vi "Dashboard Main.vi"() -> ()   [LabVIEW 2025]
uses:
  builds/FRC_Dashboard/data/Bordeaux/Types/Single Cmd Info.ctl
  <vilib>/picture/picture.llb/imagedata.ctl
  <vilib>/Rock Robotics/WPI/DriverStation/WPI_DriverStationAllianceInfo.ctl
  <vilib>/Utility/miscctls.llb/LVPoint32TypeDef.ctl
  builds/FRC_Dashboard/data/Bordeaux/Types/Drive Type.ctl
  52f2dcef-b32f-41dc-9262-467f65fbdc6c.vi
  builds/FRC_Dashboard/data/Bordeaux/Global Settings.vi
  <vilib>/Rock Robotics/Network Tables/NT Write String Array.vi
  <vilib>/Rock Robotics/WPI/Dashboard/WPI_DashboardLogging Global.vi
  <vilib>/Rock Robotics/Network Tables/NT Write Number.vi
  <vilib>/Rock Robotics/Network Tables/NT Write Boolean.vi
  <vilib>/Rock Robotics/Network Tables/NT Read Integer.vi
  <vilib>/Rock Robotics/Network Tables/NT Read Number.vi
  <vilib>/Rock Robotics/Network Tables/NT Read Numeric Array.vi
  <vilib>/ErrorRing/Error Ring.xnode
  <vilib>/MakerHub/Toolbox/LMH-Toolbox.lvlib
panel:
  out "path":string[](array[string])
  out "ACTIVITY STATUS":dbl[][](graph)
  in  "Camera Settings Right":T1={"Frame Rate"=30, "Compression"=30, "Size"=1, "DB Camera Config"=FALSE} {"Frame Rate" scale=1.0..30.0; "Compression" scale=100.0..-1.0; "Size" items=["640x480", "320x240", "160x120"]}
  in  "Camera Name Right":string(combo)="No Camera Selection"
  out "NT Connection":bool
  in  "Camera Settings":T1={"Frame Rate"=30, "Compression"=30, "Size"=1, "DB Camera Config"=FALSE} {"Frame Rate" scale=1.0..30.0; "Compression" scale=100.0..-1.0; "Size" items=["640x480", "320x240", "160x120"]}
  in  "Camera Name":string(combo)="No Camera Selection"
  in  "TCP":refnum<k5>
  in  "Rec Mode":enum32{"Stop", "Record", "Playback"}(radio)
  out "Robot IP":string
  out "Image Message":string="Timeout in Camera Communications"
  in  "Dashboard Tab":T2(tab)
  in  "Offset":dbl=270.0
  out "Boolean 2":bool
  in  "Active Status":bool
  out "Boolean":bool
  out "Picture":picture
  in  "Auto Delay?":bool
  in  "Delay Time (s)":dbl
  in  "Aquitaine File":string
  in  "Auto Calibrate":bool=TRUE
  in  "Manual Paths":string[](array[string])
  in  "Max Rotation":dbl=270.0
  in  "Max Translation":dbl=19.0
  in  "Deadband":dbl=0.05
  in  "Auto Selector":T3(ring)
  out "IMU":dbl(knob) scale=-180.0..180.0
  in  "Select Auto":string(combo)="Select Autonomous ..."
  out "Mode":T4(ring)=enum."Auto Disabled"
  out "Camera Perf":cluster{"Bandwidth (Mbps)":dbl, "FPS":dbl}
  out "Camera Perf 2":string
  out "Auto Picture":picture
  out "path info":string
  in  "restart":bool
  out "Picture 2":picture
  out "Camera Perf 3":string
  out "DISTANCE":dbl
  out "PTH":dbl(knob) scale=-180.0..180.0
  out "Tree":string(tree)
  # "HW"
  # "HW"
  # "IMU"
  # "SWERVE"
  # "AUTONOMOUS"
  # "CONFIGS"
  # "TAG VISIBILITY"
  # "STATUS"
  # "PLACEHOLDER"
  # "PLACEHOLDER"
  # "CAN ERROR"
  # "SENSOR FAULT"
  # "GATE DRIVER"
  # "No POWER"
  # "Full FORWARD"
  # "Full REVERSE"
  # "BRUSHED BRAKE"
  # "BRUSHED COAST"
  # "BRUSHLESS BRAKE"
  # "BRUSHLESS COAST"
  # "RECOVERY MODE/OFF"
  # "https://cdn8.bigcommerce.com/s-t3eo8vwp22/product_images/uploaded_images/fault-no-12v.gif"
  # "PIGEON 2"
  # "DAMAGED HARDWARE"
  # "BOOTLOADER"
  # "CAN FAULT"
  # "ROBOT DISABLED"
  # "ROBOT ENABLED"
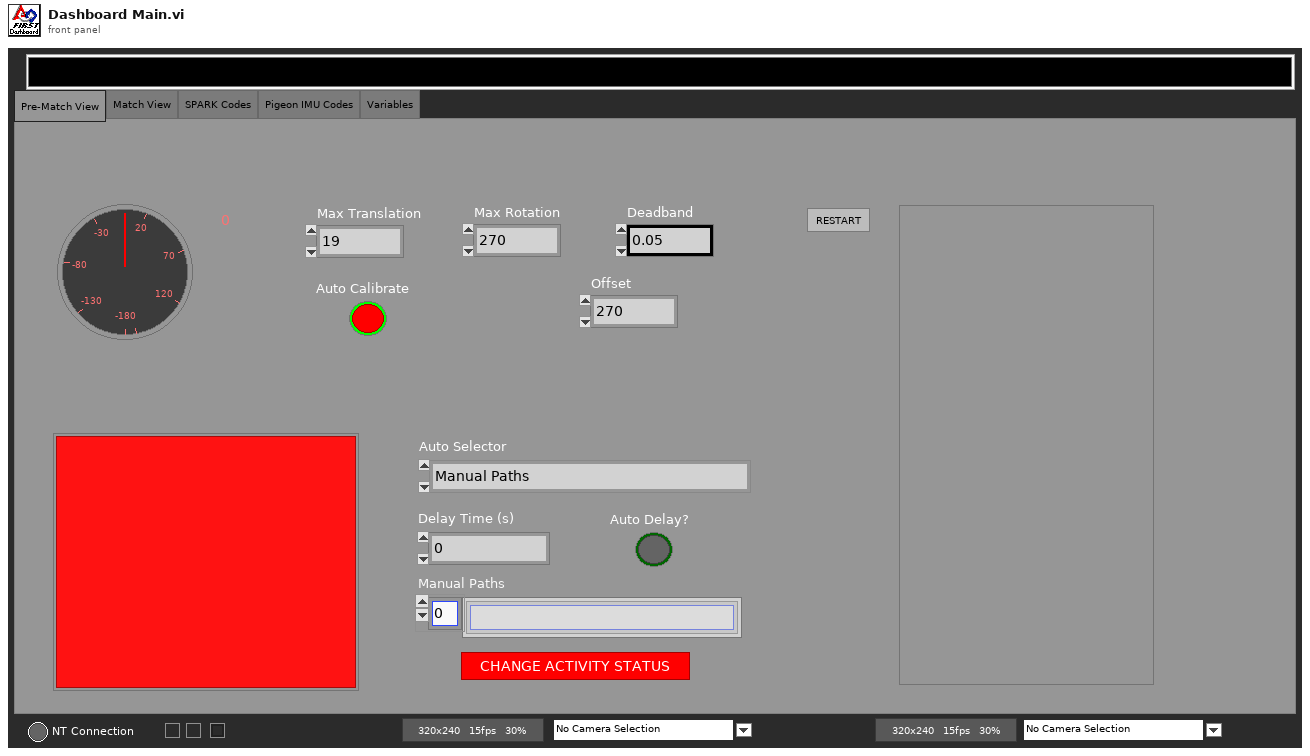
[diagram p1: front panel]
types:
  T1 = cluster{"Frame Rate":i32, "Compression":i32, "Size":u16, "DB Camera Config":bool}
  T2 = enum32{"Pre-Match View", "Match View", "SPARK Codes", "Pigeon IMU Codes", "Variables"}
  T3 = enum16{"Manual Paths", "Custom Paths", "Red Right Neutral", "Blue Right Neutral", "Red Left Neutral", "Blue Left Neutral", "Red Right 86 ", "Blue Right 86", "Red Left 86", "Blue Left 86"}
  T4 = enum8{"Tele-Op Disabled", "Tele-Op Enabled", "Auto Disabled", "Auto Enabled", "Test Disabled", "Test Enabled", "Disconnected", "No Code", "E-Stop"}
  T5 = cluster{"Save Path":path, "Interval (s)":dbl, "Keep":i32}
  T6 = typedef "Image Type" = u32
  T7 = enum32{"Pre-Match View", "Match View", "SparkMax Codes", "Pigeon IMU Codes", "Variables"}
  T8 = cluster{"IDs":cluster{"RPC field ID":u16, "Unique ID":u16}, "String":string}
  T9 = typedef "IMAQ Image.ctl" = refnum<image>
  T10 = cluster{"Dashboard Tab":refnum<vi>, "Rec Mode":refnum<vi>, "Tree":refnum<vi>, "Camera Perf 2":refnum<vi>, "Camera Settings":refnum<vi>, "Camera Name":refnum<vi>, "Camera Name":refnum<vi>}
  T11 = cluster{"Camera Name Right":string, string, "Saved DB Images Info":cluster{"Save Path":path, "Interval (s)":dbl, "Keep":i32}}
  T12 = cluster{"Global Rectangle":i32[], "Contours":cluster{"Contour Type":u32, "ROI Type":u32, "Points":i32[]}[]}
  T13 = cluster{"Camera Name":string, string, "Saved DB Images Info":cluster{"Save Path":path, "Interval (s)":dbl, "Keep":i32}}
  T14 = typedef "Single Cmd Info.ctl" = cluster{"Name":string, "CPTM.DataType":variant, "All Control Values Variant":cluster{"Name":string, "Variant Data":variant}[], "icon full":T15, "icon scaled":T15, "Path":path, "Subsystem Color":u32}
  T15 = typedef "imagedata.ctl" = cluster{"image type":i32, "image depth":i32, "image":u8[], "mask":u8[], "colors":u32[], "Rectangle":cluster{"left":i16, "top":i16, "right":i16, "bottom":i16}}
  T16 = typedef "Drive Type.ctl" = enum16{"Nonholonomic", "Holonomic"}
  T17 = typedef "LVPoint32TypeDef.ctl" = cluster{"Horizontal":i32, "Vertical":i32}
  T18 = cluster{"Index":i32, "Pt Test Results":enum16{"Miss", "Rect Hit", "Arrow Hit"}}
  T19 = cluster{"Error Strings":string, "Disable Counts":cluster{u16, u16}, "Rail Faults":cluster{u16, u16, u16}, "Robot IP":string, "DB Mode":u8, "Event Info":cluster{"Name":string, "Type":u8, "Number":u16, "Replay":u8}}
  T20 = cluster{"Storage":cluster{"Disk Free":u64, "RAM Block":u32, "RAM free":u32}, "CPU Utilization":cluster{"CPU % ISR":sgl, "CPU % Time Crit":sgl, "CPU % Timed Str":sgl, "CPU % High":sgl, "CPU % Above":sgl, "CPU % Normal":sgl, "CPU % Low":sgl}, "CAN":cluster{"% Bus Utilization":sgl, "Bus Off Cnt":u32, "TX_FIFO Full Cnt":u32, "Receive Error Cnt":u8, "Transmit Error Cnt":u8}, "HID":cluster{"HID Outputs":u32, "Rumble Low":u16, "Rumble High":u16}[]}
  T21 = cluster{"Status bits":cluster{"Test Mode":bool, "Autonomous":bool, "Enabled":bool, "Code Start":bool, "Brownout":bool, "Reserved 2":bool, "Reserved 3":bool, "E-Stop":bool}, "Code Trace":cluster{"Disabled":bool, "TeleOp":bool, "Auto":bool, "Test":bool}, "Controller Type":enum16{"unknown", "cRIO", "roboRio"}, "Code?":enum16{"unknown", "noCode", "code"}, "Battery V":dbl}
  T22 = cluster{"Control Bits":cluster{"TestMode":bool, "Autonomous":bool, "Enabled":bool, "FMS Present":bool, bool, bool, bool, "E-Stop":bool}, "Team Station ":u8, "Countdown":sgl, "Joystick Values":cluster{"Axes":dbl[], "Buttons":bool[], "POVs":i16[]}[]}
  T23 = cluster{"Robot Backwards":bool, "Reverse Path":bool}
  T24 = typedef "Trajectory Data.ctl" = cluster{"Segment Name":string, "Type":T25, "Traj Pos Points":cluster{"x":dbl, "y":dbl, "th":dbl}[], "Traj Vel Points":cluster{"V":dbl, "Omega":dbl, "V vector":cluster{"y":dbl, "x":dbl}}[], "Accel Index":i32, "Decel Index":i32}[]
  T25 = typedef "Segment Type.ctl" = enum16{"Accel Straight", "Const Straight", "Blend", "Circle", "Bezier"}
  T26 = typedef "Overrides.ctl" = cluster{"Count":string, "Angular Override":dbl, "Enabled?":bool, "Velocity Override":dbl, "Angle Override":dbl}[]
  T27 = typedef "Angluar Limits.ctl" = cluster{"Velocity (deg/s)":dbl, "Accel (deg/s^2)":dbl, "Jerk (deg/s^3)":dbl}
  T28 = cluster{"Sample Period (s)":dbl, cluster{"Velocity (fps)":dbl, "Accel (fps^2)":dbl, "Jerk (fps^3)":dbl, "StoopidFast (fps)":dbl}, "Conditions":cluster{"vInitial (fps)":dbl, "vFinal (fps)":dbl}, "Overrides":T26, "Angular Limits":T27}
  T29 = typedef "Path Type.ctl" = enum16{"Clothoid", "Bezier"}
  T30 = cluster{"status":bool, "code":bool, "source":bool}
  T31 = cluster{"Reversals":cluster{"Robot Backwards":bool, "Reverse Path":bool}, "Trajectory Data":T24, "Commands out":cluster{"Time (s)":dbl, T14, bool}[], "Fields":cluster{"Sample Period (s)":dbl, cluster{"Velocity (fps)":dbl, "Accel (fps^2)":dbl, "Jerk (fps^3)":dbl, "StoopidFast (fps)":dbl}, "Conditions":cluster{"vInitial (fps)":dbl, "vFinal (fps)":dbl}, "Overrides":T26, "Angular Limits":T27}, "Points out":cluster{"x":dbl, "y":dbl, "th":dbl}[], "Overall":cluster{"Time (s)":dbl, "Distance (ft)":dbl}, "Zero V":bool, "Trajectory Meta":cluster{"Drive Type":T16, "Path Type":T29}}
  T32 = typedef "MEGA traj.ctl" = cluster{cluster{"Robot Backwards":bool, "Reverse Path":bool}, "Trajectory Data":T24, "sorted array out":cluster{"Time (s)":dbl, T14, bool}[], cluster{"Sample Period (s)":dbl, "Limits":T33, "Conditions":cluster{"vInitial (fps)":dbl, "vFinal (fps)":dbl}, "Overrides":T26, "Angular Limits":T27}, "Updated Waypoints":cluster{"x":dbl, "y":dbl, "th":dbl}[], cluster{"Time (s)":dbl, "Distance (ft)":dbl}, "Zero Velocity":bool, cluster{"Drive Type":T16, "Path Type":T29}}[]
  T33 = typedef "Limits.ctl" = cluster{"Velocity (fps)":dbl, "Accel (fps^2)":dbl, "Jerk (fps^3)":dbl, "StoopidFast (fps)":dbl}
  T34 = cluster{"Horizontal":dbl, "Vertical":dbl, "th":dbl}
  T35 = cluster{"Horizontal":dbl, "Vertical":dbl, "th":dbl}[]
  T36 = cluster{"Operation":enum16{"Update", "Clear"}, "Color Box":u32}[]
  T37 = cluster{"Image Size":bool, "Image Type":bool, "Pixel Value":bool, "ROI Information":bool, "Zoom Factor":bool}
  T38 = cluster{"Shift":bool, "Ctrl":bool, "Alt":bool, "Cmd":bool, "Opt":bool}
  T39 = typedef "WPI_DriverStationAllianceInfo.ctl" = enum16{"Red", "Blue", "Invalid"}
  T40 = cluster{"Numeric":dbl, "Numeric":dbl, "Numeric":dbl}
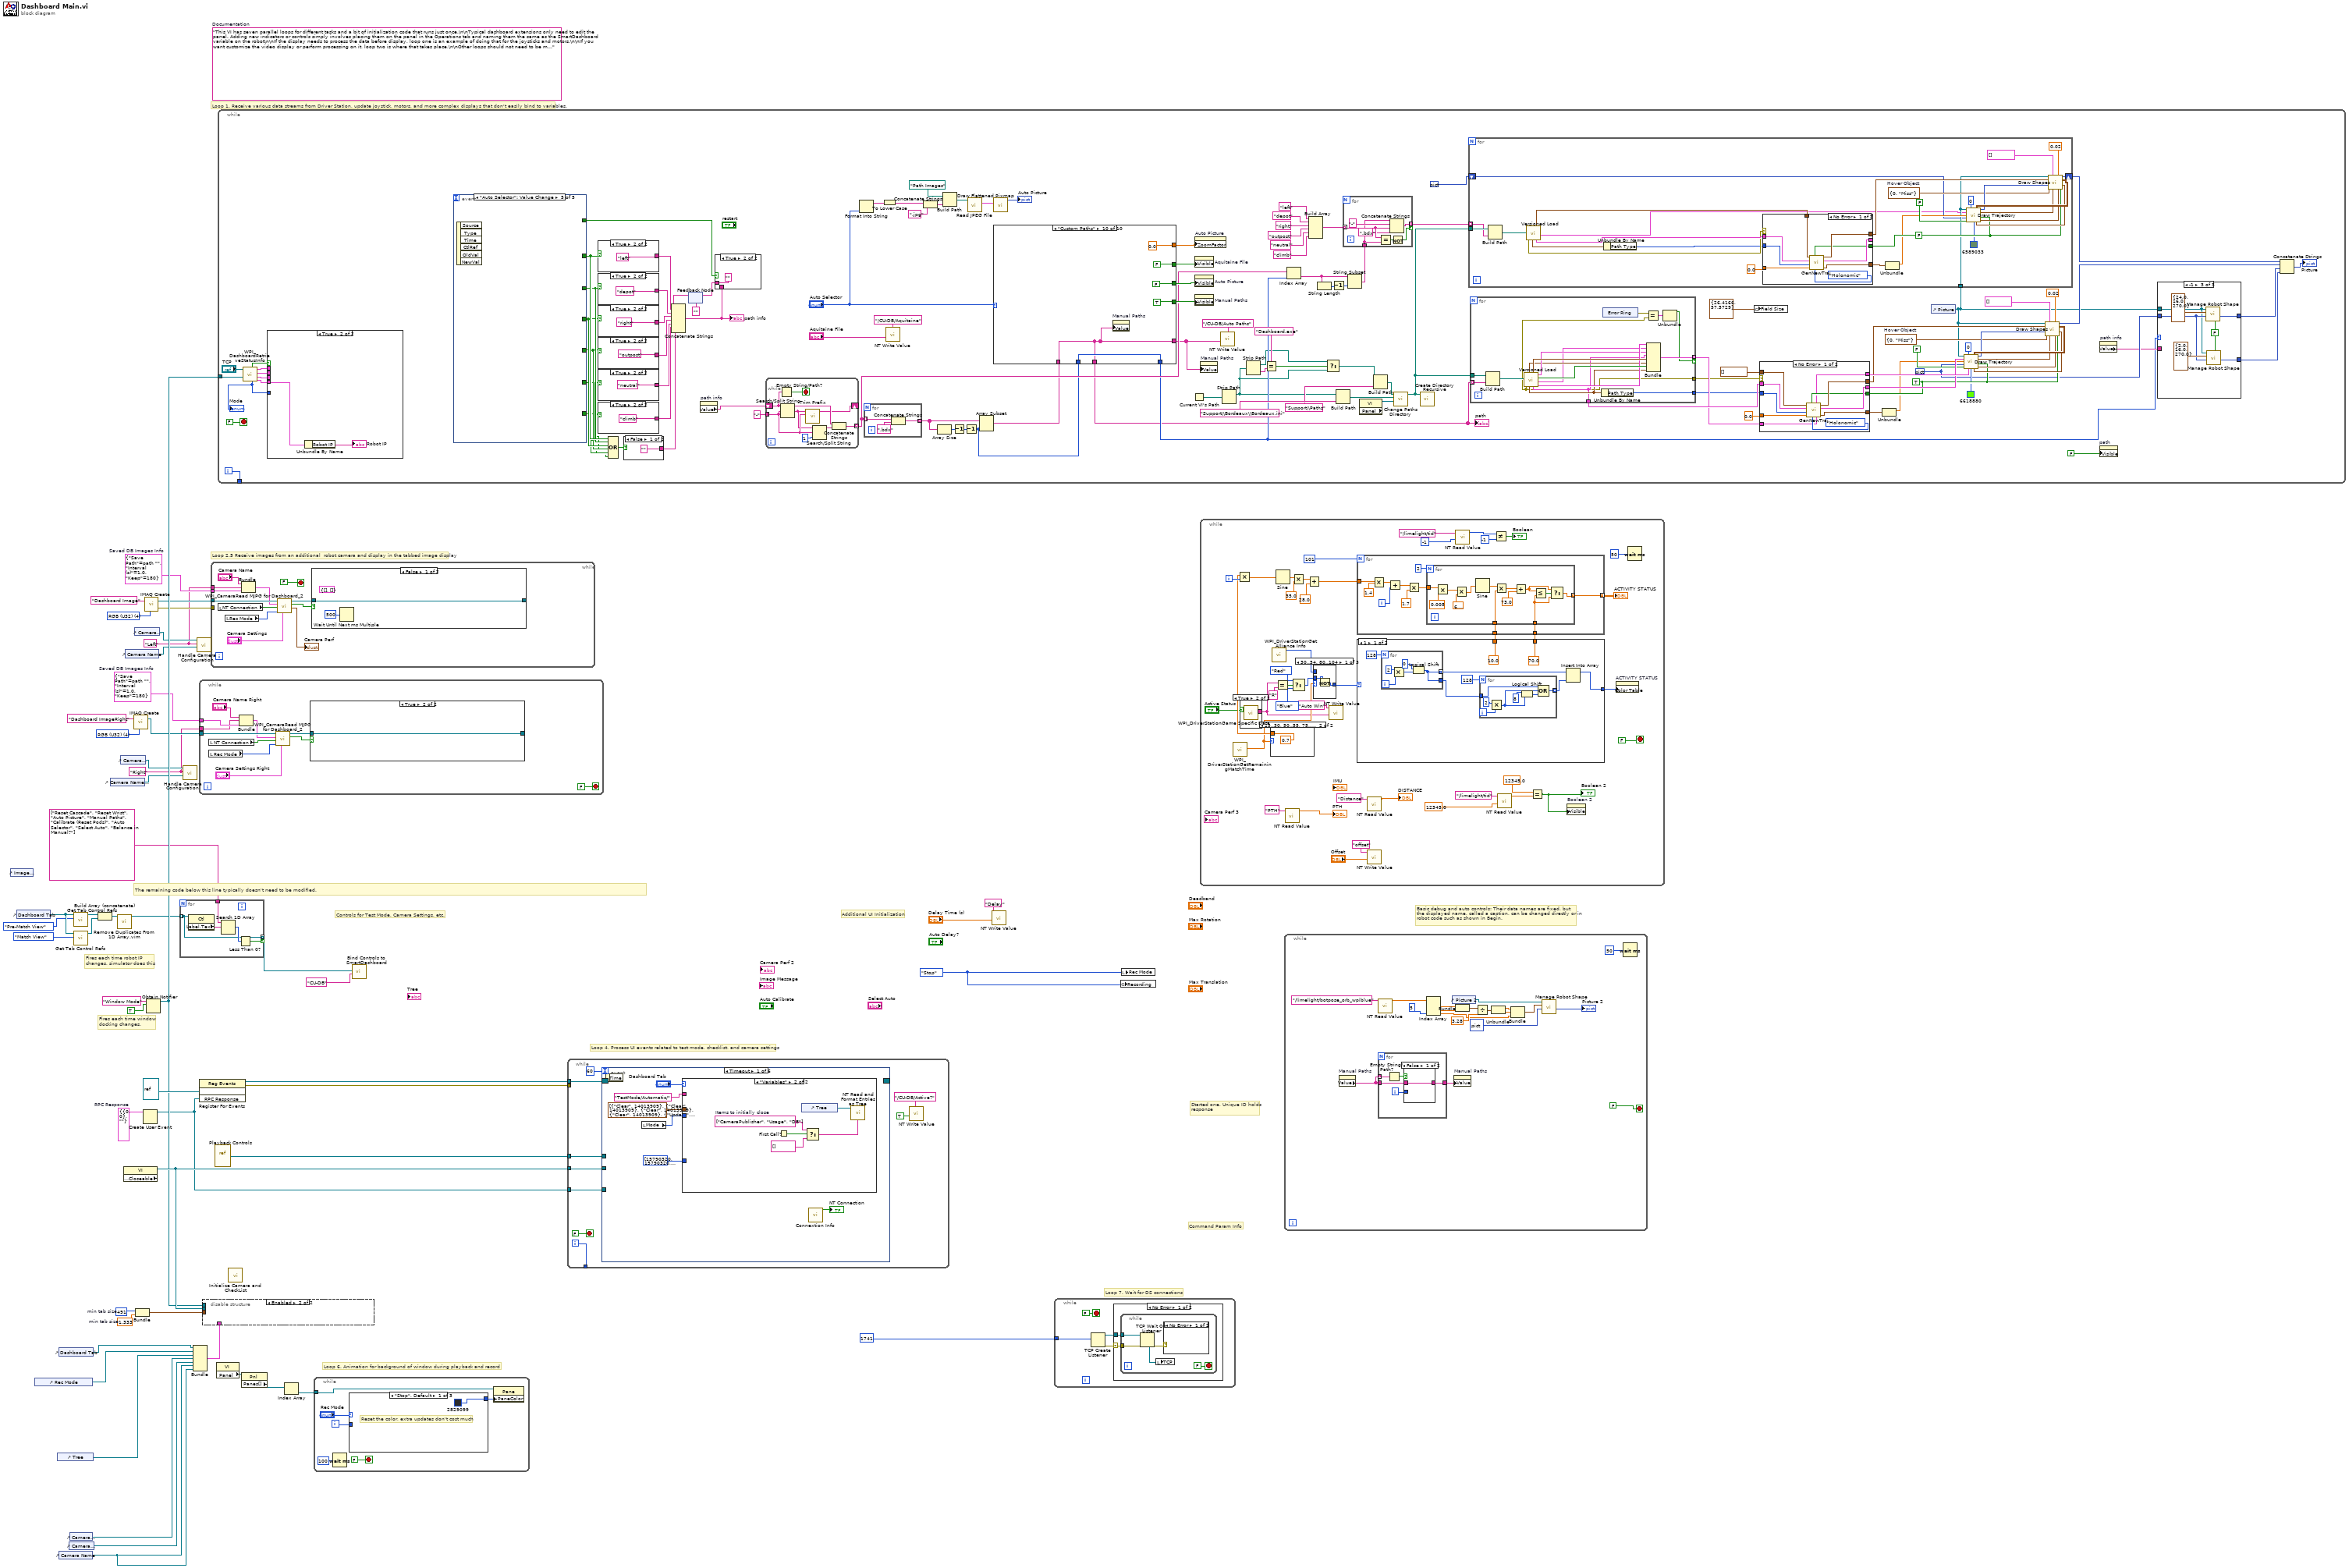
[diagram p0: block diagram]
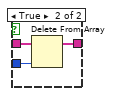
[diagram p2: hidden frame]
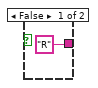
[diagram p3: hidden frame]
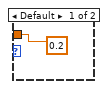
[diagram p6: hidden frame]
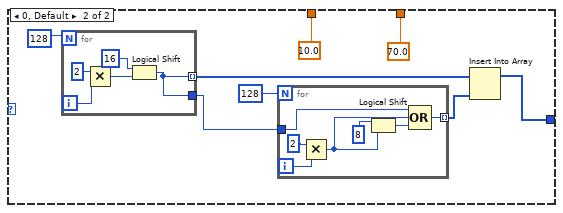
[diagram p7: hidden frame]
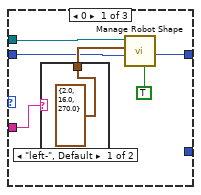
[diagram p8: hidden frame]
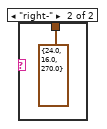
[diagram p9: hidden frame]
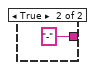
[diagram p13: hidden frame]
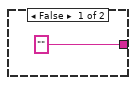
[diagram p14: hidden frame]
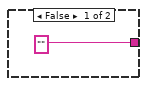
[diagram p15: hidden frame]
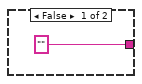
[diagram p16: hidden frame]
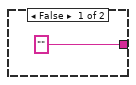
[diagram p17: hidden frame]
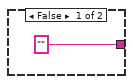
[diagram p18: hidden frame]
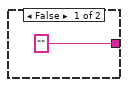
[diagram p19: hidden frame]
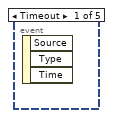
[diagram p20: hidden frame]
diagram:
  w4 = "Right"
  w9 = T5 {"Save Path"=path "", "Interval (s)"=1.0, "Keep"=180}  # Saved DB Images Info
  w11 = T6 4 items=["Grayscale (U8)", "Grayscale (I16)", "Grayscale (SGL)", "Complex (CSG)", "RGB (U32)", "HSL (U32)", "RGB (U64)"] ("Image Type")
  w27 = T5 {"Save Path"=path "", "Interval (s)"=1.0, "Keep"=180}  # Saved DB Images Info
  w8 = "Left"
  w30 = T6 4 items=["Grayscale (U8)", "Grayscale (I16)", "Grayscale (SGL)", "Complex (CSG)", "RGB (U32)", "HSL (U32)", "RGB (U64)"] ("Image Type")
  w34 = T8 {"IDs"={"RPC field ID"=0, "Unique ID"=0}, "String"=""}  # RPC Response
  w41 = 491  # min tab size
  w40 = 1.333  # min tab size
  w43 = enum32{"Stop", "Record", "Playback"}."Stop" ("Rec Mode")
  (unwired) "This VI has seven parallel loops for different tasks and a bit of initialization code that runs just once.\n\nTypical dashboard extensions only need to edit the panel. Adding new indicators or controls simply involves placing them on the panel in the Operations tab and naming them the same as the SmartDashboard variable on the robot\n\nIf the display needs to process the data before display, loop one is an example of doing that for the joysticks and motors.\n\nIf you want customize the video display or perform processing on it, loop two is where that takes place.\n\nOther loops should not need to be modified. They are pretty standard, and document the task they perform."  # Documentation
  # "Loop 2.5 Receive images from an additional  robot camera and display in the tabbed image display"
  # "Command Param Info"
  # "Started one, Unique ID holds\nresponse"
  # "Loop 7. Wait for DS connections"
  # "Basic debug and auto controls: Their data names are fixed, but\nthe displayed name, called a caption, can be changed directly or in\nrobot code such as shown in Begin."
  # "Controls for Test Mode, Camera Settings, etc."
  # "Additional UI Initialization"
  # "Loop 6. Animation for background of window during playback and record"
  # "Fires each time robot IP\nchanges, simulator does this"
  # "Fires each time window\ndocking changes."
  # "The remaining code below this line typically doesn't need to be modified."
  # "Loop 4. Process UI events related to test mode, checklist, and camera settings"
  # "Loop 1. Receive various data streams from Driver Station, update joystick, motors, and more complex displays that don't easily bind to variables."
  n1 = control-ref of="Image Message"() -> ()  [unwired: 1 out]
  n2 = control-ref of="Dashboard Tab"() -> (w25:refnum<vi>)
  n3 = control-ref of="Rec Mode"() -> (w37:refnum<vi>)
  n4 = control-ref of="Tree"() -> (w26:refnum<vi>)
  n5 = control-ref of="Camera Name"() -> (w3:refnum<vi>)
  n6 = control-ref of="Dashboard Tab"() -> (w17:refnum<vi>)
  n7 = control-ref of="Camera Settings"() -> (w28:refnum<vi>)
  n8 = control-ref of="Camera Perf 2"() -> (w32:refnum<vi>)
  n9 = call <vilib>:"Get Tab Control Refs.vi"("Page Index"=T7."Pre-Match View" ("Dashboard Tab"), "TabControl in"=w25) -> ("ControlsOnPage"=w24:refnum<vi>[])  [unwired: 9 in]
  n10 = call <vilib>:"Get Tab Control Refs.vi"("Page Index"=T7."Match View" ("Dashboard Tab"), "TabControl in"=w25) -> ("ControlsOnPage"=w23:refnum<vi>[])  [unwired: 9 in]
  n11 = Build Array (concatenate)(w24, w23) -> (w22:refnum<vi>[])
  n12 = control-ref of="Camera Name Right"() -> (w5:refnum<vi>)
  n13 = call "Remove Duplicates From 1D Array.vim"("array"=w22) -> ("array with duplicates removed"=w19:refnum<vi>[])  [unwired: 10 in]
  n14 = control-ref of="Camera Settings Right"() -> (w6:refnum<vi>)
  n15 = property class="VI" props=["Front Panel.Closeable"]() -> (reference out=w42:refnum<vi>)  [unwired: 2 in, 2 out]
  n16 = control-ref of="Camera Name"() -> (w13:refnum<vi>)
  n17 = call "IMAQ Create"("Image Name"="Dashboard ImageRight", "Image Type"=w11) -> ("New Image"=w7:T9)  [unwired: 2 in, 2 out]
  n18 = control-ref of="Camera Settings"() -> (w14:refnum<vi>)
  n19 = Bundle("min tab size"=w41, "min tab size"=w40) -> (w39:cluster{"min tab size":i32, "min tab size":dbl})  [unwired: 1 in]
  n20 = Create User Event(user event datatype=w34) -> (user event=w33:refnum<user-event>)  [unwired: 1 in, 1 out]
  n21 = call "IMAQ Create"("Image Name"="Dashboard Image", "Image Type"=w30) -> ("New Image"=w12:T9, "error out"=w29:errorcluster)  [unwired: 2 in, 1 out]
  n22 = Obtain Notifier(name (unnamed)="Window Mode", notification data type=TRUE) -> (notifier out=w36:refnum<notifier>)  [unwired: 2 in, 2 out]
  n23 = for {
    tunnel: string[] ["Reset Cascade", "Reset Wrist", "Auto Picture", "Manual Paths", "Calibrate (Reset Pods)", "Auto Selector", "Select Auto", "Balance in Manual?"] -> [w57]
    tunnel: w19 -> [w54] mode=indexing
    tunnel: [w54] -> w18 mode=indexing if=w53
    n24 = property class="Ctl"(reference=w54) -> ("Label.Text"=w56:string)  [unwired: 1 in, 2 out]
    n25 = Search 1D Array(1D array=w57, element=w56) -> (index of element=w55:i32)  [unwired: 1 in]
    n26 = Less Than 0?(x=w55) -> (x < 0?=w53:bool)
  }
  n27 = call "Handle Camera Configuration.vi"("CameraNameRef"=w5, "Display Name"=w4, "ClusterRef"=w6) -> ()  [unwired: 9 in]
  n28 = Bundle("Dashboard Tab"=w17, "Rec Mode"=w37, "Tree"=w26, "Camera Perf 2"=w32, "Camera Settings"=w28, "Camera Name"=w3, "Camera Name"=w3) -> (w38:T10)  [unwired: 1 in]
  n29 = call "Handle Camera Configuration.vi"("CameraNameRef"=w13, "Display Name"=w8, "ClusterRef"=w14) -> ()  [unwired: 9 in]
  n30 = while {
    tunnel: w9 -> [w62]
    tunnel: w7 -> [w65]
    tunnel: w4 -> [w59]
    stop <- FALSE stop-if-true
    n31 = local read "NT Connection"() -> (w64:bool)
    n32 = local read "Rec Mode"() -> (w63:enum32{"Stop", "Record", "Playback"})
    n33 = Bundle("Camera Name Right"="Camera Name Right", w59, "Saved DB Images Info"=w62) -> (w58:T11)  [unwired: 1 in]
    n34 = call <vilib>:"WPI_CameraRead MJPG for Dashboard_2.vi"("Camera Settings"="Camera Settings Right", "Rec Mode"=w63, "NT Connection"=w64, "Capture Info"=w58, "Image in"=w65) -> ("Active"=w67:bool, "Image\\ out"=w68:T9)  [unwired: 4 in, 1 out]
    n35 = case shown="True" w67 {
      tunnel: w68 -> [w69 w71]
      tunnel: [w69 w71] -> _
      frame False {
        (unwired) T12 {"Global Rectangle"=[], "Contours"=[]} ("ROI")
        n36 = Wait Until Next ms Multiple(millisecond multiple=u32 500) -> ()  [unwired: 1 out]
      }
      frame True {
      }
    }
  }
  n37 = register-events(refnum<vi> refnum, w33) -> (reference out=w46:refnum<event-registration>, error out=w45:errorcluster)  [unwired: 2 in]
  n38 = disable-structure shown="Enabled" {
    disable-tunnel: w42 -> [_ _]
    disable-tunnel: w39 -> [_ _]
    disable-tunnel: w38 -> [_ _]
    disable-tunnel: w36 -> [_ _]
    frame Disabled {
      # "Loop 5. Adjusts placement onscreen, hides the titlebar, etc."
    }
    frame Enabled {
    }
  }
  n39 = while {
    tunnel: w12 -> [w83]
    tunnel: w29 -> [_]
    tunnel: w27 -> [w73]
    tunnel: w8 -> [w75]
    stop <- FALSE stop-if-true
    n40 = local read "NT Connection"() -> (w74:bool)
    n41 = local read "Rec Mode"() -> (w72:enum32{"Stop", "Record", "Playback"})
    n42 = Bundle("Camera Name"="Camera Name", w75, "Saved DB Images Info"=w73) -> (w78:T13)  [unwired: 1 in]
    n43 = call <vilib>:"WPI_CameraRead MJPG for Dashboard_2.vi"("Camera Settings"="Camera Settings", "Rec Mode"=w72, "NT Connection"=w74, "Capture Info"=w78, "Image in"=w83) -> ("perf info"=→"Camera Perf":cluster{"Bandwidth (Mbps)":dbl, "fps":dbl}, "Active"=w79:bool, "Image\\ out"=w81:T9)  [unwired: 4 in]
    n44 = case shown="False" w79 {
      tunnel: w81 -> [w84 w86]
      tunnel: [w84 w86] -> _
      frame False {
        (unwired) T12 {"Global Rectangle"=[], "Contours"=[]} ("ROI")
        n45 = Wait Until Next ms Multiple(millisecond multiple=u32 500) -> ()  [unwired: 1 out]
      }
      frame True {
      }
    }
  }
  n46 = vi-ref "Playback Controls.vi"() -> (w47:refnum<vi>)
  n47 = property class="VI"() -> ("Panel"=w49:refnum<vi>)  [unwired: 2 in, 2 out]
  n48 = while {
    tunnel: [w200] -> _
    tunnel: w36 -> [w193]
    i -> [w200]
    stop <- FALSE stop-if-true
    w162 = TRUE ("MEGA?")
    w163 = T18 {"Index"=0, "Pt Test Results"=enum."Miss"}  # Hover Object
    w100 = picture data[5B] ("new picture")
    n49 = call <vilib>:"WPI_DashboardRetrieveStatusInfo.vi"("Window Mode Notifier"=w193, "TCP Cnx"="TCP") -> ("Power and Errors"=w195:T19, "Robot Metrics"=w198:T20, "Status Info"=w199:T21, "Control Info"=w196:T22, "Robot Mode"=w177:T4, "Process?"=w197:bool)  [unwired: 4 in]
    "Mode" <- w177
    n50 = case shown="True" w197 {
      tunnel: w199 -> [_ _]
      tunnel: w198 -> [_ _]
      tunnel: w196 -> [_ _]
      tunnel: w195 -> [_ w360]
      tunnel: w177 -> [_ _]
      frame False {
        n51 = Wait (ms)(milliseconds to wait=u32 20) -> ()  [unwired: 1 out]
      }
      frame True {
        n52 = Unbundle By Name(w360) -> ("Robot IP"=→"Robot IP":string)
      }
    }
    n53 = event shown="[4] \"Auto Selector\": Value Change" {
      selector: _ -> [_ _ _ _ _]
      dyn-events: _ -> [_ _ _ _ _]
      timeout: _ -> [_ _ _ _ _]
      tunnel: [_ w295 _ w328 _] -> w135
      tunnel: [_ w294 _ w328 _] -> w134
      tunnel: [_ w293 _ w328 _] -> w133
      tunnel: [_ w292 _ w328 _] -> w132
      tunnel: [_ w291 _ w328 _] -> w131
      tunnel: [_ w290 _ w328 _] -> w130
      tunnel: [_ _ _ TRUE _] -> w123
      event Timeout {
        n54 = event-data() -> ()  [unwired: 1 in, 3 out]
      }
      event "Picture": Mouse Down {
        n55 = event-data() -> ("Coords"=w314:T17)  [unwired: 1 in, 7 out]
        n56 = In Range and Coerce(upper limit=T17 {"Horizontal"=-520, "Vertical"=110}, x=w314, lower limit=T17 {"Horizontal"=-560, "Vertical"=70}) -> (In Range?=w313:cluster{"Horizontal":bool, "Vertical":bool})  [unwired: 1 out]
        n57 = In Range and Coerce(upper limit=T17 {"Horizontal"=-480, "Vertical"=230}, x=w314, lower limit=T17 {"Horizontal"=-520, "Vertical"=190}) -> (In Range?=w308:cluster{"Horizontal":bool, "Vertical":bool})  [unwired: 1 out]
        n58 = In Range and Coerce(upper limit=T17 {"Horizontal"=-290, "Vertical"=110}, x=w314, lower limit=T17 {"Horizontal"=-330, "Vertical"=70}) -> (In Range?=w305:cluster{"Horizontal":bool, "Vertical":bool})  [unwired: 1 out]
        n59 = In Range and Coerce(upper limit=T17 {"Horizontal"=-310, "Vertical"=230}, x=w314, lower limit=T17 {"Horizontal"=-350, "Vertical"=190}) -> (In Range?=w302:cluster{"Horizontal":bool, "Vertical":bool})  [unwired: 1 out]
        n60 = In Range and Coerce(upper limit=T17 {"Horizontal"=-340, "Vertical"=50}, x=w314, lower limit=T17 {"Horizontal"=-500, "Vertical"=-80}) -> (In Range?=w299:cluster{"Horizontal":bool, "Vertical":bool})  [unwired: 1 out]
        n61 = In Range and Coerce(upper limit=T17 {"Horizontal"=-415, "Vertical"=220}, x=w314, lower limit=T17 {"Horizontal"=-435, "Vertical"=200}) -> (In Range?=w296:cluster{"Horizontal":bool, "Vertical":bool})  [unwired: 1 out]
        n62 = Unbundle(w299) -> ("Horizontal"=w301:bool, "Vertical"=w300:bool)
        n63 = Unbundle(w296) -> ("Horizontal"=w298:bool, "Vertical"=w297:bool)
        n64 = Unbundle(w313) -> ("Horizontal"=w312:bool, "Vertical"=w311:bool)
        n65 = Unbundle(w302) -> ("Horizontal"=w304:bool, "Vertical"=w303:bool)
        n66 = Unbundle(w308) -> ("Horizontal"=w310:bool, "Vertical"=w309:bool)
        n67 = Unbundle(w305) -> ("Horizontal"=w307:bool, "Vertical"=w306:bool)
        n68 = And(x=w301, y=w300) -> (x .and. y?=w291:bool)
        n69 = And(x=w298, y=w297) -> (x .and. y?=w290:bool)
        n70 = And(x=w312, y=w311) -> (x .and. y?=w295:bool)
        n71 = And(x=w304, y=w303) -> (x .and. y?=w292:bool)
        n72 = And(x=w310, y=w309) -> (x .and. y?=w294:bool)
        n73 = And(x=w307, y=w306) -> (x .and. y?=w293:bool)
      }
      event "Manual Paths", "Boolean": Value Change {
        n74 = event-data() -> ()  [unwired: 1 in, 6 out]
      }
      event "restart": Value Change {
        w328 = FALSE
        n75 = event-data() -> ()  [unwired: 1 in, 6 out]
      }
      event "Auto Selector": Value Change {
        n76 = event-data() -> ()  [unwired: 1 in, 6 out]
      }
    }
    n77 = case shown="True" w135 {
      tunnel: ["" "left"] -> w154
      frame False {
      }
      frame True {
      }
    }
    n78 = case shown="True" w134 {
      tunnel: ["" "depot"] -> w153
      frame False {
      }
      frame True {
      }
    }
    n79 = case shown="True" w133 {
      tunnel: ["" "right"] -> w152
      frame False {
      }
      frame True {
      }
    }
    n80 = case shown="True" w132 {
      tunnel: ["" "outpost"] -> w151
      frame False {
      }
      frame True {
      }
    }
    n81 = case shown="True" w131 {
      tunnel: ["" "neutral"] -> w150
      frame False {
      }
      frame True {
      }
    }
    n82 = case shown="True" w130 {
      tunnel: ["" "climb"] -> w149
      frame False {
      }
      frame True {
      }
    }
    n83 = Compound Arithmetic op=OR(w135, w134, w133, w132, w131, w130) -> (w129:bool)
    n84 = case shown="False" w129 {
      tunnel: ["" ("string") "-" ("string")] -> w128
      frame False {
      }
      frame True {
      }
    }
    n85 = feedback #1("") -> (w148:string)
    n86 = Concatenate Strings(w148, w154, w153, w152, w151, w150, w149, w128) -> (w124:string)
    "path info" <- w124
    n87 = property on="path info" class="Str"() -> ("Value"=w126:string)  [unwired: 2 in, 2 out]
    n88 = case shown="True" w123 {
      tunnel: [w262 "" ("path info")] -> w125
      tunnel: w124 -> [w262 _]
      frame False {
      }
      frame True {
      }
    }
    n89 = feedback-in #1(w125) -> ()
    n90 = while {
      tunnel: "-" ("string") -> [w274]
      tunnel: [w276] -> w106 mode=indexing
      shift-right: [w275] -> _
      shift-left: w126 -> [w272]
      stop <- w273 stop-if-true
      n91 = Empty String/Path?(string/path=w272) -> (empty?=w273:bool)
      n92 = Search/Split String(string=w272, search string/char (-)=w274) -> (substring before match=w277:string, match + rest of string=w271:string)  [unwired: 1 in, 1 out]
      n93 = call <vilib>:"Trim Prefix.vi"("Prefix"=w274, "String"=w271) -> ("String"=w275:string)  [unwired: 9 in]
      n94 = Search/Split String(string=w271, search string/char (-)=w274, offset (0)=1) -> (substring before match=w269:string)  [unwired: 2 out]
      n95 = Concatenate Strings(w277, w269) -> (w276:string)
    }
    n96 = Format Into String("Auto Selector") -> (resulting string=w183:string)  [unwired: 3 in, 1 out]
    n97 = for {
      tunnel: w106 -> [w268] mode=indexing
      tunnel: [w266] -> w118 mode=indexing
      n98 = Concatenate Strings(w268, ".bdx" ("string")) -> (w266:string)
    }
    n99 = To Lower Case(string=w183) -> (all lower case string=w184:string)
    n100 = call-poly <vilib>:"NT Write Value.vi"("value"="Aquitaine File", "name"="/CU-DB/Aquitaine") -> ()  [unwired: 9 in, 1 out]
    n101 = Concatenate Strings(w184, ".jpg" ("string")) -> (w185:string)
    n102 = Array Size(array=w118) -> (size(s)=w140:i32)
    n103 = Build Path(base path=path "Path Images", name or relative path=w185) -> (appended path=w188:path)
    n104 = Decrement(x=w140) -> (x-1=w117:i32)
    n105 = Decrement(x=w117) -> (x-1=w94:i32)
    n106 = call <vilib>:"Read JPEG File.vi"("path to JPEG file"=w188) -> ("image data"=w187:T15)  [unwired: 8 in, 2 out]
    n107 = Array Subset(array=w118, length=w94) -> (w95:string[])  [unwired: 1 in]
    n108 = call <vilib>:"Draw Flattened Pixmap.vi"("image data"=w187) -> ("new picture"=→"Auto Picture":picture)  [unwired: 8 in]
    n109 = case shown="\"Custom Paths\"" "Auto Selector" {
      tunnel: ["Manual Paths" string[] ["neutral-1-FAST-LEFT.bdx", "neutral-2-FAST-LEFT.bdx", "neutral-3-FAST-LEFT.bdx", "neutral-4-FAST-LEFT.bdx", "neutral-5a-FAST-LEFT.bdx", "neutral-5b-FAST-LEFT.bdx", "neutral-6-FAST-LEFT.bdx", "neutral-7-FAST-LEFT.bdx"] ("Manual Paths") string[] ["86-1-RIGHT-V2.bdx", "86-2-RIGHT-V3.bdx", "86-3-RIGHT.bdx", "86-4-RIGHT.bdx", "86-5-RIGHT.bdx", "86-6-RIGHT.bdx", "86-7-RIGHT.bdx"] ("Manual Paths") string[] ["86-1-RIGHT-BLUE-V2.bdx", "86-2-RIGHT-BLUE-V3.bdx", "86-3-RIGHT-BLUE.bdx", "86-4-RIGHT-BLUE.bdx", "86-5-RIGHT-BLUE.bdx", "86-6-RIGHT-BLUE.bdx", "86-7-RIGHT-BLUE.bdx"] ("Manual Paths") string[] ["86-1-LEFT-V2.bdx", "86-2-LEFT-V3.bdx", "86-3-LEFT.bdx", "86-4-LEFT.bdx", "86-5-LEFT.bdx", "86-6-LEFT.bdx", "86-7-LEFT.bdx"] ("Manual Paths") string[] ["86-1-LEFT-BLUE-V2.bdx", "86-2-LEFT-BLUE-V3.bdx", "86-3-LEFT-BLUE.bdx", "86-4-LEFT-BLUE.bdx", "86-5-LEFT-BLUE.bdx", "86-6-LEFT-BLUE.bdx", "86-7-LEFT-BLUE.bdx"] ("Manual Paths") string[] ["neutral-1-FAST-LEFT-BLUE.bdx", "neutral-2-FAST-LEFT-BLUE.bdx", "neutral-3-FAST-LEFT-BLUE.bdx", "neutral-4-FAST-LEFT-BLUE.bdx", "neutral-5a-FAST-LEFT-BLUE.bdx", "neutral-5b-FAST-LEFT-BLUE.bdx", "neutral-6-FAST-LEFT-BLUE.bdx", "neutral-7-FAST-LEFT-BLUE.bdx"] ("Manual Paths") string[] ["neutral-1-FAST-RIGHT.bdx", "neutral-2-FAST-RIGHT.bdx", "neutral-3-FAST-RIGHT.bdx", "neutral-4-FAST-RIGHT.bdx", "neutral-5a-FAST-RIGHT.bdx", "neutral-5b-FAST-RIGHT.bdx", "neutral-6-FAST-RIGHT.bdx", "neutral-7-FAST-RIGHT.bdx"] ("Manual Paths") string[] ["neutral-1-FAST-RIGHT-BLUE.bdx", "neutral-2-FAST-RIGHT-BLUE.bdx", "neutral-3-FAST-RIGHT-BLUE.bdx", "neutral-4-FAST-RIGHT-BLUE.bdx", "neutral-5a-FAST-RIGHT-BLUE.bdx", "neutral-5b-FAST-RIGHT-BLUE.bdx", "neutral-6-FAST-RIGHT-BLUE.bdx", "neutral-7-FAST-RIGHT-BLUE.bdx"] ("Manual Paths") w423] -> w91
      tunnel: [FALSE ("Visible") FALSE ("Visible") FALSE ("Visible") FALSE ("Visible") FALSE ("Visible") FALSE ("Visible") FALSE ("Visible") FALSE ("Visible") FALSE ("Visible") FALSE ("Visible")] -> w192
      tunnel: [TRUE ("Visible") TRUE ("Visible") TRUE ("Visible") TRUE ("Visible") TRUE ("Visible") TRUE ("Visible") TRUE ("Visible") TRUE ("Visible") TRUE ("Visible") TRUE ("Visible")] -> w179
      tunnel: [FALSE ("Visible") FALSE ("Visible") FALSE ("Visible") FALSE ("Visible") FALSE ("Visible") FALSE ("Visible") FALSE ("Visible") FALSE ("Visible") FALSE ("Visible") FALSE ("Visible")] -> w189
      tunnel: [sgl 0.0 ("Zoom Factor") sgl 0.0 ("Zoom Factor") sgl 0.0 ("Zoom Factor") sgl 0.0 ("Zoom Factor") sgl 0.0 ("Zoom Factor") sgl 0.0 ("Zoom Factor") sgl 0.0 ("Zoom Factor") sgl 0.0 ("Zoom Factor") sgl 0.0 ("Zoom Factor") sgl 0.0 ("Zoom Factor")] -> w176
      tunnel: w95 -> [_ _ _ _ _ _ _ _ _ w423]
      tunnel: w94 -> [_ _ _ _ _ _ _ _ _ w424]
      tunnel: [-2 -2 -2 -2 -2 -2 -2 -2 -2 w424] -> w93
      tunnel: ["Manual Paths" string[] ["left-neutral.bdx", "neutral-leftpreload.bdx", "leftpreload-neutral.bdx", "neutral-leftbump.bdx"] ("Manual Paths") string[] ["left-neutral.bdx", "neutral-leftpreload.bdx", "leftpreload-neutral.bdx", "neutral-leftbump.bdx"] ("Manual Paths") string[] ["left-neutral.bdx", "neutral-leftpreload.bdx", "leftpreload-neutral.bdx", "neutral-leftbump.bdx"] ("Manual Paths") string[] ["left-neutral.bdx", "neutral-leftpreload.bdx", "leftpreload-neutral.bdx", "neutral-leftbump.bdx"] ("Manual Paths") string[] ["left-neutral.bdx", "neutral-leftpreload.bdx", "leftpreload-neutral.bdx", "neutral-leftbump.bdx"] ("Manual Paths") string[] ["left-neutral.bdx", "neutral-leftpreload.bdx", "leftpreload-neutral.bdx", "neutral-leftbump.bdx"] ("Manual Paths") string[] ["right-neutral.bdx", "neutral-rightpreload.bdx", "rightpreload-neutral.bdx", "neutral-rightbump.bdx"] ("Manual Paths") string[] ["right-neutral.bdx", "neutral-rightpreload.bdx", "rightpreload-neutral.bdx", "neutral-rightbump.bdx"] ("Manual Paths") w423] -> w92
      frame "Manual Paths", Default {
      }
      frame "Red Left Neutral" {
      }
      frame "Red Right 86 " {
      }
      frame "Blue Right 86" {
      }
      frame "Red Left 86" {
      }
      frame "Blue Left 86" {
      }
      frame "Blue Left Neutral" {
      }
      frame "Red Right Neutral" {
      }
      frame "Blue Right Neutral" {
      }
      frame "Custom Paths" {
        n110 = property on="Manual Paths" class="Arr (strict)"("Value"=w423) -> ()  [unwired: 2 in, 2 out]
      }
    }
    "path" <- w92
    n111 = Current VI's Path() -> (path=w139:path)
    n112 = property on="Auto Picture" class="Pict"("ZoomFactor"=w176) -> ()  [unwired: 2 in, 2 out]
    n113 = property on="Aquitaine File" class="Str"("Visible"=w189) -> ()  [unwired: 2 in, 2 out]
    n114 = property on="Auto Picture" class="Pict"("Visible"=w192) -> ()  [unwired: 2 in, 2 out]
    n115 = property on="Manual Paths" class="Arr (strict)"("Visible"=w179) -> ()  [unwired: 2 in, 2 out]
    n116 = property on="Manual Paths" class="Arr (strict)"("Value"=w91) -> ()  [unwired: 2 in, 2 out]
    n117 = call-poly <vilib>:"NT Write Value.vi"("value"=w91, "name"="/CU-DB/Auto Paths") -> ()  [unwired: 9 in, 1 out]
    n118 = Strip Path(path=w139) -> (stripped path=w89:path)  [unwired: 1 out]
    n119 = Strip Path(path=w89) -> (stripped path=w90:path, name=w138:string)
    n120 = Equal?(x="Dashboard.exe", y=w138) -> (x = y?=w88:bool)
    n121 = Index Array(array=w106, index=w93) -> (element=w104:string)
    n122 = Build Array("left", "depot", "right", "outpost", "neutral", "climb") -> (w108:string[])
    n123 = String Length(string=w104) -> (length=w103:i32)
    n124 = Select(t=w90, s=w88, f=w89) -> (s? t:f=w87:path)
    n125 = Decrement(x=w103) -> (x-1=w102:i32)
    n126 = Build Path(base path=w89, name or relative path="Support\\Bordeaux\\Bordeaux.ini" ("format string")) -> (appended path=w144:path)
    n127 = String Subset(string=w104, length (rest)=w102) -> (substring=w105:string)  [unwired: 1 in]
    n128 = for {
      tunnel: w108 -> [w222] mode=indexing
      tunnel: w105 -> [w221]
      tunnel: [w223] -> w107 mode=indexing if=w219
      n129 = Equal?(x=w222, y=w221) -> (x = y?=w220:bool)
      n130 = Concatenate Strings(w221, "-" ("string"), w222, ".bdx" ("string")) -> (w223:string)
      n131 = Not(x=w220) -> (.not. x?=w219:bool)
    }
    n132 = property class="VI" props=["Panel"]() -> (reference out=w146:refnum<vi>)  [unwired: 2 in, 2 out]
    n133 = Build Path(base path=w87, name or relative path="Support\\Paths" ("format string")) -> (appended path=w136:path)
    n134 = call "Change Paths Directory.vi"("VI Refnum"=w146, "config path"=w144, "Bordeaux paths directory"=w136) -> ("Bordeaux paths out"=w116:path)  [unwired: 8 in]
    n135 = call <vilib>:"Create Directory Recursive.vi"("directory"=w116) -> ()  [unwired: 4 in, 3 out]
    n136 = for {
      tunnel: [w355] -> w169
      tunnel: [w343] -> w170
      tunnel: [w348] -> w173 mode=indexing if=w345
      tunnel: [w346] -> w174
      tunnel: w116 -> [w341]
      tunnel: w92 -> [w340] mode=indexing
      n137 = Build Path(base path=w341, name or relative path=w340) -> (appended path=w356:path)
      n138 = call "Versioned Load.vi"("path"=w356) -> ("Reversals"=w352:T23, "Trajectory Data"=w347:T24, "Zero V"=w354:bool, "Commands out"=w351:cluster{"Time (s)":dbl, T14, bool}[], "Fields"=w346:T28, "Points out"=w353:cluster{"x":dbl, "y":dbl, "th":dbl}[], "Trajectory Meta"=w349:cluster{"Drive Type":T16, "Path Type":T29}, "Overall"=w350:cluster{"Time (s)":dbl, "Distance (ft)":dbl}, "error out"=w343:errorcluster)  [unwired: 2 in]
      n139 = Unbundle By Name(w349) -> ("Path Type"=w355:T29)
      n140 = xnode "Error Ring"() -> ("error out"=w344:errorcluster)
      n141 = Equal?(x=w344, y=w343) -> (x = y?=w342:T30)
      n142 = Bundle("Reversals"=w352, "Trajectory Data"=w347, "Commands out"=w351, "Fields"=w346, "Points out"=w353, "Overall"=w350, "Zero V"=w354, "Trajectory Meta"=w349) -> (w348:T31)  [unwired: 1 in]
      n143 = Unbundle(w342) -> ("status"=w345:bool)  [unwired: 2 out]
    }
    n144 = global write "Global Settings.vi" "Field Size"(cluster{"width":dbl, "height":dbl} {"width"=26.4166, "height"=57.5729} ("Field Size")) -> ()
    n145 = case shown="No Error" w170 {
      tunnel: cluster{"x":dbl, "y":dbl, "th":dbl}[] [] ("Points out") -> [w339 _]
      tunnel: 0.0 ("Stoopid Overlap %") -> [w338 _]
      tunnel: [w336 _] -> w167
      tunnel: [w335 _] -> w168
      tunnel: w169 -> [w334 _]
      tunnel: w174 -> [w333 _]
      tunnel: w162 -> [w332 _]
      tunnel: w173 -> [w331 _]
      tunnel: [w330 _] -> w175
      tunnel: [w329 _] -> w142
      frame No Error {
        n146 = call "GenNewTraj.vi"("MEGA traj"=w331, "Drive Type"=Drive_Type."Holonomic", "MEGA?"=w332, "Stoopid Overlap %"=w338, "Path Type"=w334, "Parameters"=w333, "Points in"=w339) -> ("Time & Dist"=w329:cluster{"Time (s)":dbl, "Distance (ft)":dbl}, "Trajectory Data"=w336:T24, "Updated Waypoints"=w335:cluster{"x":dbl, "y":dbl, "th":dbl}[], "MEGA traj 2"=w330:T32)  [unwired: 1 out]
      }
      frame Error {
      }
    }
    n147 = Unbundle(w142) -> ("Time (s)"=w141:dbl)  [unwired: 1 out]
    n148 = control-ref of="Picture"() -> (w99:refnum<vi>)
    n149 = for {
      tunnel: w99 -> [w234]
      tunnel: w116 -> [w229]
      shift-right: [w233] -> w122
      shift-left: picture data[5B] ("new picture") -> [w228]
      tunnel: w107 -> [w227] mode=indexing
      w242 = FALSE ("MEGA?")
      w243 = T18 {"Index"=0, "Pt Test Results"=enum."Miss"}  # Hover Object
      n150 = Build Path(base path=w229, name or relative path=w227) -> (appended path=w231:path)
      n151 = call "Versioned Load.vi"("path"=w231) -> ("Trajectory Data"=w225:T24, "Fields"=w252:T28, "Points out"=w226:cluster{"x":dbl, "y":dbl, "th":dbl}[], "Trajectory Meta"=w230:cluster{"Drive Type":T16, "Path Type":T29}, "error out"=w249:errorcluster)  [unwired: 2 in, 4 out]
      n152 = Unbundle By Name(w230) -> ("Path Type"=w248:T29)
      n153 = case shown="No Error" w249 {
        tunnel: 0.0 ("Stoopid Overlap %") -> [w261 _]
        tunnel: [w259 _] -> _
        tunnel: [w258 _] -> w247
        tunnel: w248 -> [w257 _]
        tunnel: w252 -> [w256 _]
        tunnel: w242 -> [w255 _]
        tunnel: [w254 _] -> w236
        tunnel: w226 -> [w253 _]
        frame No Error {
          n154 = call "GenNewTraj.vi"("Drive Type"=Drive_Type."Holonomic", "MEGA?"=w255, "Stoopid Overlap %"=w261, "Path Type"=w257, "Parameters"=w256, "Points in"=w253) -> ("Time & Dist"=w254:cluster{"Time (s)":dbl, "Distance (ft)":dbl}, "Trajectory Data"=w259:T24, "Updated Waypoints"=w258:cluster{"x":dbl, "y":dbl, "th":dbl}[])  [unwired: 1 in, 2 out]
        }
        frame Error {
        }
      }
      n155 = Unbundle(w236) -> ("Time (s)"=w235:dbl)  [unwired: 1 out]
      n156 = call "Draw Trajectory.vi"("Picture in"=w234, "Robot Index"=0, "Trajectory Data"=w225, "time"=w235, "new picture in"=w228, "MEGA?"=w242, "Hide Path"=FALSE, "color(black)"=u32 6589033) -> ("Path Points MEGA"=w251:cluster{"x":dbl, "y":dbl}[][], "new picture"=w246:picture, "Output Point"=w245:T34, "Output Point MEGA"=w250:T35, "Path Points"=w244:cluster{"x":dbl, "y":dbl}[])  [unwired: 3 in]
      n157 = call "Draw Shapes.vi"("Picture in"=w234, "Commands"=cluster{"Time (s)":dbl, T14, "Enabled":bool}[] [], "Sample Period (s)"=0.02, "Points"=w247, "Path Points MEGA"=w251, "new picture in"=w246, "Output Point MEGA"=w250, "Results"=w243, "Output Point"=w245, "Path Points"=w244, "MEGA?"=w242) -> ("new picture out"=w233:picture)  [unwired: 4 in]
    }
    n158 = call "Draw Trajectory.vi"("Picture in"=w99, "Robot Index"=0, "Trajectory Data"=w167, "time"=w141, "new picture in"=w100, "MEGA?"=w162, "Hide Path"=FALSE, "MEGA traj"=w175, "color(black)"=u32 6618880) -> ("Path Points MEGA"=w172:cluster{"x":dbl, "y":dbl}[][], "new picture"=w166:picture, "Output Point"=w165:T34, "Output Point MEGA"=w171:T35, "Path Points"=w164:cluster{"x":dbl, "y":dbl}[])  [unwired: 2 in]
    n159 = call "Draw Shapes.vi"("Picture in"=w99, "Commands"=cluster{"Time (s)":dbl, T14, "Enabled":bool}[] [], "Sample Period (s)"=0.02, "Points"=w168, "Path Points MEGA"=w172, "new picture in"=w166, "Output Point MEGA"=w171, "Results"=w163, "Output Point"=w165, "Path Points"=w164, "MEGA?"=w162) -> ("new picture out"=w121:picture)  [unwired: 4 in]
    n160 = property on="path" class="Arr (strict)"("Visible"=FALSE) -> ()  [unwired: 2 in, 2 out]
    n161 = property on="path info" class="Str"() -> ("Value"=w96:string)  [unwired: 2 in, 2 out]
    n162 = case shown="-1" w93 {
      tunnel: [w204 w210 w217] -> w101
      tunnel: w100 -> [w203 w210 w213]
      tunnel: w99 -> [w205 _ w212]
      tunnel: [_ w210 w211] -> w98
      tunnel: w96 -> [w202 _ _]
      frame 0 {
        n163 = case shown="\"left-\", Default" w202 {
          tunnel: [cluster{"x":dbl, "y":dbl, "th":dbl} {"x"=2.0, "y"=16.0, "th"=270.0} ("Robot Position (ft)") cluster{"x":dbl, "y":dbl, "th":dbl} {"x"=24.0, "y"=16.0, "th"=270.0} ("Robot Position (ft)")] -> w207
          frame "left-", Default {
          }
          frame "right-" {
          }
        }
        n164 = call "Manage Robot Shape.vi"("Lighter"=TRUE, "new picture in"=w203, "Robot Position (ft)"=w207, "Pict Ref"=w205) -> ("new picture out"=w204:picture)  [unwired: 5 in, 2 out]
      }
      frame Default {
      }
      frame -1 {
        w215 = FALSE ("Lighter")
        n165 = call "Manage Robot Shape.vi"("Lighter"=w215, "new picture in"=w213, "Robot Position (ft)"=cluster{"x":dbl, "y":dbl, "th":dbl} {"x"=24.0, "y"=16.0, "th"=270.0}, "Pict Ref"=w212) -> ("new picture out"=w217:picture)  [unwired: 5 in, 2 out]
        n166 = call "Manage Robot Shape.vi"("Lighter"=w215, "new picture in"=w213, "Robot Position (ft)"=cluster{"x":dbl, "y":dbl, "th":dbl} {"x"=2.0, "y"=16.0, "th"=270.0}, "Pict Ref"=w212) -> ("new picture out"=w211:picture)  [unwired: 5 in, 2 out]
      }
    }
    n167 = Concatenate Strings(w122, w121, w101, w98) -> (→"Picture":picture)
  }
  n168 = call "Initialize Camera and CheckList.vi"() -> ()  [unwired: 12 in]
  n169 = property class="Pnl"(reference=w49) -> ("Panes[]"=w50:refnum<vi>[])  [unwired: 1 in, 2 out]
  n170 = Index Array(array=w50) -> (element=w48:refnum<vi>)  [unwired: 1 in]
  n171 = while {
    tunnel: w48 -> [w430]
    i -> [w433]
    stop <- FALSE stop-if-true
    n172 = Wait (ms)(milliseconds to wait=u32 100) -> ()  [unwired: 1 out]
    n173 = case shown="\"Stop\", Default" "Rec Mode" {
      tunnel: w433 -> [_ _ w448]
      tunnel: [u32 2829099 ("Base Color") u32 11141120 ("Target Color") w437] -> w429
      frame "Stop", Default {
        # "Reset the color, extra updates don't cost much"
      }
      frame "Record" {
      }
      frame "Playback" {
        # "Playback"
        n174 = Quotient & Remainder(x=w448, y=u32 50 ("milliseconds to wait")) -> (x-y*floor(x/y)=w444:u32)  [unwired: 1 out]
        n175 = Divide(x=w444, y=u32 100 ("milliseconds to wait")) -> (x/y=w441:dbl)
        n176 = Multiply(x=6.283185307179586, y=w441) -> (x*y=w446:dbl)
        n177 = Sine(x=w446) -> (sin(x)=w445:dbl)
        n178 = Absolute Value(x=w445) -> (abs(x)=w438:dbl)
        n179 = call "Interpolate RGB Color.vi"("Proportion"=w438, "Target Color"=u32 30976, "Base Color"=u32 2829099) -> ("Result Color"=w437:u32)  [unwired: 8 in]
      }
    }
    n180 = property class="Pane"(reference=w430, "PaneColor"=w429) -> ()  [unwired: 1 in, 2 out]
  }
  n181 = call <vilib>:"Bind Controls to SmartDashboard.vi"("Path Prefix"="CU-DB", "Bound Control Refs"=w18) -> ()  [unwired: 10 in]
  n182 = while {
    tunnel: [w455] -> _
    tunnel: w47 -> [w454]
    tunnel: w46 -> [w453]
    tunnel: w45 -> [_]
    tunnel: w42 -> [w452]
    tunnel: w33 -> [w451]
    i -> [w455]
    stop <- FALSE stop-if-true
    n183 = event shown="[0] Timeout" {
      selector: w453 -> [_ _ _ _ _ _]
      dyn-events: [_ _ _ w477 _ _] -> _
      timeout: u32 60 ("milliseconds to wait") -> [_ _ _ _ _ _]
      tunnel: w454 -> [_ _ _ w479 w494 _]
      tunnel: w452 -> [_ _ _ w475 _ _]
      tunnel: w451 -> [_ _ _ w473 _ _]
      event Timeout {
        n184 = event-data() -> ()  [unwired: 1 in, 1 out]
        n185 = local read "Mode"() -> (w460:T4)
        n186 = case shown="\"Variables\"" "Dashboard Tab" {
          tunnel: "TestMode/Automatic/" ("Name Pattern") -> [_ _]
          tunnel: T36 [{"Operation"=enum."Clear", "Color Box"=14013909}, {"Operation"=enum."Clear", "Color Box"=14013909}, {"Operation"=enum."Clear", "Color Box"=14013909}, {"Operation"=enum."Clear", "Color Box"=14013909}, {"Operation"=enum."Update", "Color Box"=14013909}, {"Operation"=enum."Update", "Color Box"=16777215}, {"Operation"=enum."Clear", "Color Box"=14013909}, {"Operation"=enum."Clear", "Color Box"=14013909}, {"Operation"=enum."Clear", "Color Box"=14013909}] -> [_ _]
          tunnel: w460 -> [_ _]
          tunnel: u32[] [15790320, 15790320, 15790320, 15790320, 16777215, 16777215, 15790320, 15790320, 15790320] -> [_ _]
          frame Default {
          }
          frame "Variables" {
            w466 = string[] ["CameraPublisher", "Usage", "DB"]  # Items to initially close
            n187 = First Call?() -> (First Call?: T/F=w467:bool)
            n188 = control-ref of="Tree"() -> (w468:refnum<vi>)
            n189 = Select(t=w466, s=w467, f=string[] []) -> (s? t:f=w464:string[])
            n190 = call <vilib>:"NT Read and Format Entries as Tree.vi"("Tags to  Close"=w464, "Tree Refnum"=w468) -> ()  [unwired: 8 in, 2 out]
          }
        }
        n191 = call <vilib>:"Connextion Info.vi"() -> ("Connected"=→"NT Connection":bool)  [unwired: 10 in, 1 out]
      }
      event "Select Auto": Mouse Enter {
        # "Populate the combo box with the list of autonomous options"
        n192 = event-data() -> ()  [unwired: 1 in, 1 out]
        n193 = call <vilib>:"NT Read String Array.vi"("name"="Auto List" ("Name")) -> ("value"=w469:string[])  [unwired: 8 in, 2 out]
        n194 = property on="Select Auto" class="CmbBox"("Strings[]"=w469) -> ()  [unwired: 2 in, 2 out]
      }
      event "Select Auto": Value Change {
        # "User modified the Auto Selection. Write to NT variable so robot knows."
        n195 = event-data() -> ("NewVal"=w471:string)  [unwired: 1 in]
        n196 = call <vilib>:"NT Write String.vi"("value"=w471, "name"="Auto Selector" ("Name")) -> ()  [unwired: 9 in, 1 out]
      }
      event "Rec Mode": Value Change {
        # "Update globals for recording mode and path to read log from.\nClear when logging and let NetworkTables set path for vision to\nuse."
        n197 = event-data() -> ("NewVal"=w480:enum32{"Stop", "Record", "Playback"})  [unwired: 1 in]
        n198 = global write "WPI_DashboardLogging Global.vi" "Logging Filename"(path "") -> ()
        n199 = global write "WPI_DashboardLogging Global.vi" "Recording"(w480) -> ()
        n200 = case shown="\"Playback\"" w480 {
          tunnel: w479 -> [_ w482 w491]
          tunnel: [_ _ w490] -> w477
          tunnel: [_ _ w489] -> _
          tunnel: w475 -> [_ _ w487]
          tunnel: cluster{i32, i32} {0, 340} -> [_ _ w486]
          tunnel: [_ _ T37 {"Image Size"=TRUE, "Image Type"=TRUE, "Pixel Value"=TRUE, "ROI Information"=TRUE, "Zoom Factor"=FALSE} ("Image Information Shown:All Elements")] -> _
          tunnel: [_ _ TRUE ("Zoom Factor")] -> _
          tunnel: w473 -> [_ _ w483]
          frame Default {
          }
          frame "Stop", "Record" {
            # "Place Window too"
            n201 = invoke class="VI" method="FP.Close"(reference=w482) -> (reference out=w481:refnum<vi>)  [unwired: 2 in, 2 out]
            n202 = invoke class="VI" method="Abort VI"(reference=w481) -> ()  [unwired: 2 in, 3 out]
          }
          frame "Playback" {
            n203 = call "Open Playback Panel.vi"("Offset"=w486, "DB VI Ref"=w487, "Playback in"=w491) -> ("Playback out"=w488:refnum<vi>)  [unwired: 8 in]
            n204 = register-events(w488, w483) -> (reference out=w490:refnum<event-registration>, error out=w489:errorcluster)  [unwired: 2 in]
          }
        }
        n205 = call <vilib>:"WPI_DashboardNT Log FieldName Cache.vi"("Operation"=enum16{"Lookup/Add", "Index", "Clear"}."Clear") -> ()  [unwired: 8 in, 3 out]
      }
      event Panel Close {
        # "Abort playback window and ourself"
        n206 = event-data() -> ()  [unwired: 1 in, 4 out]
        n207 = invoke class="VI" method="FP.Close"(reference=w494) -> (reference out=w493:refnum<vi>)  [unwired: 2 in, 2 out]
        n208 = invoke class="VI" method="Abort VI"(reference=w493) -> (error out=w492:errorcluster)  [unwired: 2 in, 2 out]
        n209 = invoke class="VI" method="Abort VI"(error in=w492) -> ()  [unwired: 2 in, 3 out]
      }
      event "Tree": Double Click {
        n210 = event-data() -> ("PlatMods"=w500:T38, "Tag"=w497:string)  [unwired: 1 in]
        n211 = Unbundle(w500) -> ("Shift"=w499:bool)  [unwired: 4 out]
        n212 = String Subset(string=w497, length (rest)=1 ("length (rest)")) -> (substring=w496:string)  [unwired: 1 in]
        n213 = Not(x=w499) -> (.not. x?=w498:bool)
        n214 = case shown="\"/\"" w496 {
          tunnel: w497 -> [_ w502]
          tunnel: w498 -> [_ w501]
          frame Default {
          }
          frame "/" {
            n215 = call <vilib>:"NT Update Persistence.vi"("Persistence"=w501, "Name"=w502) -> ()  [unwired: 9 in, 1 out]
          }
        }
      }
    }
    n216 = call-poly <vilib>:"NT Write Value.vi"("value"=TRUE ("Boolean"), "name"="/CU-DB/Active?" ("Name")) -> ()  [unwired: 9 in, 1 out]
  }
  n217 = call-poly <vilib>:"NT Write Value.vi"("value"="Delay Time (s)", "name"="Delay") -> ()  [unwired: 9 in, 1 out]
  n218 = while {
    tunnel: u16 1741 ("timeout ms (25000)") -> [w504]
    stop <- FALSE stop-if-true
    n219 = TCP Create Listener(10:w504) -> (0:w503:errorcluster, 3:w505:refnum<k5>)  [unwired: 4 in, 1 out]
    n220 = case shown="No Error" w503 {
      selector: w503 -> [w507 _]
      tunnel: w505 -> [w508 _]
      frame No Error {
        n221 = while {
          tunnel: w508 -> [w511]
          tunnel: w507 -> [w510]
          stop <- FALSE stop-if-true
          n222 = TCP Wait On Listener(8:w510, 11:w511) -> (0:w512:errorcluster, 4:w513:refnum<k5>)  [unwired: 2 in, 3 out]
          n223 = local write "TCP"(w513) -> ()
          n224 = case shown="No Error" w512 {
            frame No Error {
            }
            frame Error {
              n225 = Wait (ms)(milliseconds to wait=u32 1000) -> ()  [unwired: 1 out]
            }
          }
        }
      }
      frame Error {
        n226 = Wait (ms)(milliseconds to wait=u32 1000) -> ()  [unwired: 1 out]
      }
    }
  }
  n227 = global write "WPI_DashboardLogging Global.vi" "Recording"(w43) -> ()
  n228 = local write "Rec Mode"(w43) -> ()
  n229 = while {
    i -> [w551]
    stop <- FALSE stop-if-true
    n230 = call <vilib>:"WPI_DriverStationGetRemainingMatchTime.vi"() -> ("Match Time(s)"=w536:sgl)  [unwired: 10 in, 1 out]
    n231 = case shown="True" "Active Status" {
      tunnel: ["R" ("Game Specific Data") w559] -> w532
      frame False {
      }
      frame True {
        n232 = call <vilib>:"WPI_DriverStationGame Specific Data.vi"() -> ("Game Specific Data"=w559:string)  [unwired: 11 in]
      }
    }
    n233 = case shown="25..30, 50..55, 75..80, 100..105, 125..130" w536 {
      tunnel: [0.2 0.7] -> w541
      frame Default {
      }
      frame 25..30, 50..55, 75..80, 100..105, 125..130 {
      }
    }
    n234 = Multiply(x=w541, y=w551) -> (x*y=w552:dbl)
    n235 = call <vilib>:"WPI_DriverStationGet Alliance Info.vi"() -> ("Alliance"=w535:T39)  [unwired: 6 in, 5 out]
    n236 = Equal?(x=w532, y="R") -> (x = y?=w543:bool)
    n237 = Sine(x=w552) -> (sin(x)=w554:dbl)
    n238 = call-poly <vilib>:"NT Read Value.vi"("name"="PTH") -> ("value"=→"PTH":dbl)  [unwired: 8 in, 2 out]
    n239 = Select(t=WPI_DriverStationAllianceInfo."Red", s=w543, f=WPI_DriverStationAllianceInfo."Blue") -> (s? t:f=w538:T39)
    n240 = Multiply(x=w554, y=35.0) -> (x*y=w550:dbl)
    n241 = Add(x=w550, y=28.0) -> (x+y=w548:dbl)
    n242 = case shown="30..54, 80..104" w536 {
      tunnel: w538 -> [w560 _ w563]
      tunnel: [w561 w562 w563] -> w537
      tunnel: w535 -> [_ w562 _]
      frame 30..54, 80..104 {
        n243 = Not(x=w560) -> (.not. x?=w561:u16)
      }
      frame Default {
      }
      frame 55..79, 105..129 {
      }
    }
    n244 = call-poly <vilib>:"NT Write Value.vi"("value"=w532, "name"="Auto Win") -> ()  [unwired: 9 in, 1 out]
    n245 = case shown="1" w537 {
      tunnel: [w569 w588] -> w544
      tunnel: [10.0 ("y") 10.0 ("y")] -> w547
      tunnel: [70.0 ("y") 70.0 ("y")] -> w546
      frame 1 {
        n246 = for {
          N: 128 -> [_]
          tunnel: [w584] -> w571 mode=indexing
          tunnel: [w584] -> w573
          i -> [w583]
          n247 = Multiply(x=2, y=w583) -> (x*y=w582:i32)
          n248 = Logical Shift(y=i16 0, x=w582) -> (x << y=w584:i32)
        }
        n249 = for {
          N: 128 -> [_]
          tunnel: w573 -> [w579]
          tunnel: [w578] -> w570 mode=indexing
          i -> [w576]
          n250 = Multiply(x=2, y=w576) -> (x*y=w575:i32)
          n251 = Logical Shift(y=i16 8, x=w575) -> (x << y=w580:i32)
          n252 = Compound Arithmetic op=OR(w579, w575, w580) -> (w578:i32)
        }
        n253 = Insert Into Array(array=w571, new element=w570) -> (w569:i32[])  [unwired: 1 in]
      }
      frame 0, Default {
        n254 = for {
          N: 128 -> [_]
          tunnel: [w604] -> w590 mode=indexing
          tunnel: [w604] -> w592
          i -> [w603]
          n255 = Multiply(x=2, y=w603) -> (x*y=w602:i32)
          n256 = Logical Shift(y=i16 16, x=w602) -> (x << y=w604:i32)
        }
        n257 = for {
          N: 128 -> [_]
          tunnel: w592 -> [w599]
          tunnel: [w598] -> w589 mode=indexing
          i -> [w596]
          n258 = Multiply(x=2, y=w596) -> (x*y=w595:i32)
          n259 = Logical Shift(y=i16 8, x=w595) -> (x << y=w600:i32)
          n260 = Compound Arithmetic op=OR(w599, w595, w600) -> (w598:i32)
        }
        n261 = Insert Into Array(array=w590, new element=w589) -> (w588:i32[])  [unwired: 1 in]
      }
    }
    n262 = for {
      N: 101 -> [_]
      tunnel: [w615] -> w545 mode=indexing
      tunnel: w548 -> [w610]
      tunnel: w547 -> [w607]
      tunnel: w546 -> [w606]
      i -> [w616]
      n263 = Multiply(x=w610, y=1.4) -> (x*y=w609:dbl)
      n264 = Add(x=w609, y=w616) -> (x+y=w612:dbl)
      n265 = Multiply(x=w612, y=1.7) -> (x*y=w613:dbl)
      n266 = for {
        N: 2 -> [_]
        tunnel: [w624] -> w615 mode=indexing
        tunnel: w613 -> [w619]
        tunnel: w607 -> [w618]
        tunnel: w606 -> [w617]
        n267 = Multiply(x=w619, y=0.005) -> (x*y=w622:dbl)
        n268 = Multiply(x=w622, y=6.283185307179586) -> (x*y=w621:dbl)
        n269 = Sine(x=w621) -> (sin(x)=w629:dbl)
        n270 = Multiply(x=w629, y=w618) -> (x*y=w628:dbl)
        n271 = Add(x=w628, y=73.0) -> (x+y=w625:dbl)
        n272 = Less Or Equal?(x=w625, y=w617) -> (x <= y?=w626:bool)
        n273 = Select(t=w625, s=w626, f=w617) -> (s? t:f=w624:dbl)
      }
    }
    "ACTIVITY STATUS" <- w545
    n274 = call-poly <vilib>:"NT Read Value.vi"("name"="Distance") -> ("value"=→"DISTANCE":dbl)  [unwired: 8 in, 2 out]
    n275 = call-poly <vilib>:"NT Write Value.vi"("value"="Offset", "name"="offset") -> ()  [unwired: 9 in, 1 out]
    n276 = call-poly <vilib>:"NT Read Value.vi"("default value"=i64 -1, "name"="/limelight/tid") -> ("value"=w531:i64)  [unwired: 7 in, 2 out]
    n277 = Not Equal?(x=w531, y=i64 -1) -> (x != y?=→"Boolean":bool)
    n278 = call-poly <vilib>:"NT Read Value.vi"("default value"=12345.0, "name"="/limelight/tid") -> ("value"=w525:dbl)  [unwired: 7 in, 2 out]
    n279 = Equal?(x=12345.0, y=w525) -> (x = y?=w519:bool)
    "Boolean 2" <- w519
    n280 = property on="Boolean 2" class="Bool (strict)"("Visible"=w519) -> ()  [unwired: 2 in, 2 out]
    n281 = property on="ACTIVITY STATUS" class="IntGraph (strict)"("Color Table"=w544) -> ()  [unwired: 2 in, 2 out]
    n282 = Wait (ms)(milliseconds to wait=u32 50) -> ()  [unwired: 1 out]
  }
  n283 = while {
    stop <- FALSE stop-if-true
    n284 = property on="Manual Paths" class="Arr (strict)"() -> ("Value"=w630:string[])  [unwired: 2 in, 2 out]
    n285 = for {
      tunnel: w630 -> [w651] mode=indexing
      tunnel: w630 -> [w652]
      tunnel: [w649] -> w631
      i -> [w653]
      n286 = Empty String/Path?(string/path=w651) -> (empty?=w650:bool)
      n287 = case shown="False" w650 {
        tunnel: w653 -> [_ w657]
        tunnel: w652 -> [w654 w656]
        tunnel: [w654 w655] -> w649
        frame False {
        }
        frame True {
          n288 = Delete From Array(array=w656, index=w657) -> (array with subset deleted=w655:string[])  [unwired: 1 in, 1 out]
        }
      }
    }
    n289 = call-poly <vilib>:"NT Read Value.vi"("name"="/limelight/botpose_orb_wpiblue") -> ("value"=w643:dbl[])  [unwired: 8 in, 2 out]
    n290 = Index Array(array=w643, index #3=5 ("index")) -> (element #1=w642:dbl, element #2=w641:dbl, element #3=w633:dbl)  [unwired: 2 in]
    n291 = control-ref of="Picture 2"() -> (w645:refnum<vi>)
    n292 = property on="Manual Paths" class="Arr (strict)"("Value"=w631) -> ()  [unwired: 2 in, 2 out]
    n293 = Bundle("Numeric"=w642, "Numeric"=w641) -> (w639:cluster{"Numeric":dbl, "Numeric":dbl})  [unwired: 1 in]
    n294 = Divide(x=w639, y=3.28) -> (x/y=w635:cluster{"Numeric":dbl, "Numeric":dbl})
    n295 = Unbundle(w635) -> ("Numeric"=w636:dbl, "Numeric"=w634:dbl)
    n296 = Bundle("Numeric"=w636, "Numeric"=w634, "Numeric"=w633) -> (w632:T40)  [unwired: 1 in]
    n297 = call "Manage Robot Shape.vi"("new picture in"=picture data[5B], "Robot Position (ft)"=w632, "Pict Ref"=w645) -> ("new picture out"=→"Picture 2":picture)  [unwired: 6 in, 2 out]
    n298 = Wait (ms)(milliseconds to wait=u32 50) -> ()  [unwired: 1 out]
  }
